vi "Joystick 2 ArmCurlSystem.vi"(10 "Secondary Joystick Buttons":bool[](array[boolean]), 11 "Secondary Joystick Values":dbl[](array[numeric])) -> (0 "Reset Arm Encoders":bool, 1 "ElbowMotor":bool, 2 "ShoulderMotor":bool, 3 "Curl Speed":dbl, 5 "Axis 4":dbl)   [LabVIEW 2018]
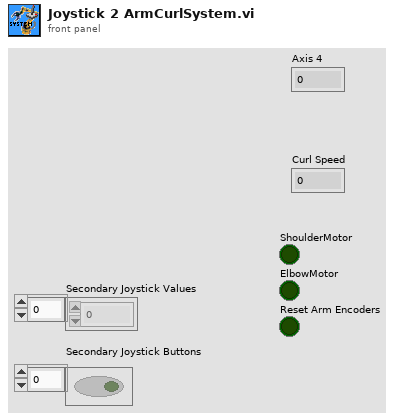
[diagram p1: front panel]
types:
  T1 = typedef "SecondaryJoystickButtons.ctl" = cluster{"Intake":bool, "Outtake":bool, "ShoulderMotor":bool, "ElbowMotor":bool, "Open Grip":bool, "Close Grip":bool, "Reset Arm Encoders":bool, "Eject Disc":bool}
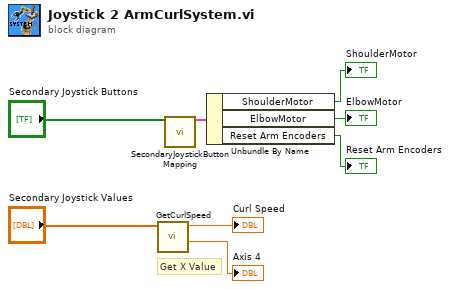
[diagram p0: block diagram]
diagram:
  # "Get X Value"
  n1 = call "GetCurlSpeed.vi"("SecondaryJoystickValues"="Secondary Joystick Values") -> ("Axis 4"=→"Axis 4":dbl, "Curl Speed"=→"Curl Speed":dbl)  [unwired: 9 in]
  n2 = call "SecondaryJoystickButtonMapping.vi"("Secondary joystick buttons"="Secondary Joystick Buttons") -> ("SecondaryJoystickButtons"=w6:T1)  [unwired: 13 in, 1 out]
  n3 = Unbundle By Name(w6) -> ("ShoulderMotor"=→"ShoulderMotor":bool, "ElbowMotor"=→"ElbowMotor":bool, "Reset Arm Encoders"=→"Reset Arm Encoders":bool)
